vi "GCOMM Close.vi"(8 "error in":errorcluster, 11 "session in":T1) -> (0 "error out":errorcluster, 3 "session out":T1)   [LabVIEW 2013]
doc: "Opens generic COM port multiplexer."
uses:
  GCOMM Session.ctl
  GCOMM Signal.ctl
  GCOMM Virtual Channel.ctl
  GCOMM Logic State.ctl
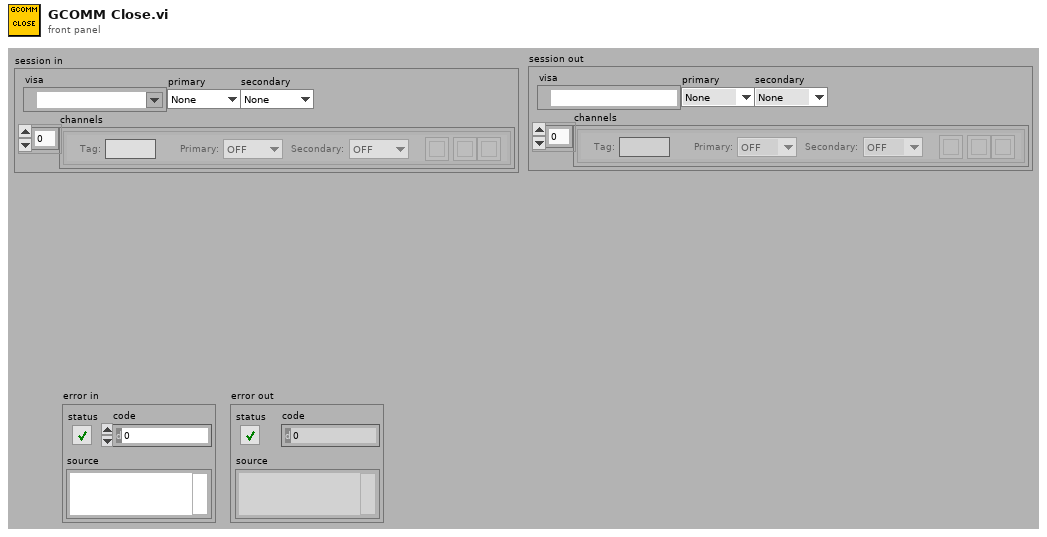
[diagram p1: front panel]
types:
  T1 = typedef "GCOMM Session.ctl" = cluster{"visa":refnum<visa-resource-name>, "primary":T2, "secondary":T2, "channels":T3[]}
  T2 = typedef "GCOMM Signal.ctl" = enum16{"None", "DTR", "RTS"}
  T3 = typedef "GCOMM Virtual Channel.ctl" = cluster{"Primary:":T4, "Secondary:":T4, "btn clr":bool, "btn up":bool, "btn down":bool, "Tag:":string}
  T4 = typedef "GCOMM Logic State.ctl" = enum16{"OFF", "ON"}
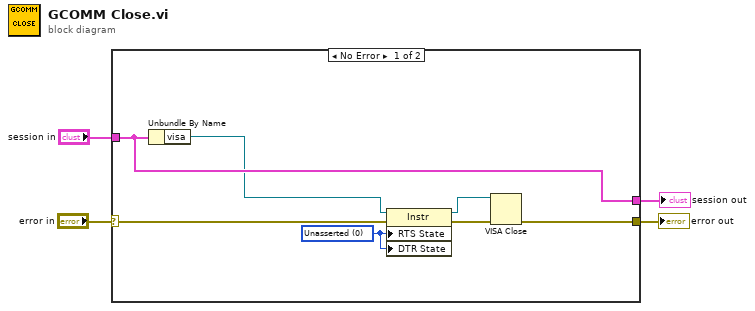
[diagram p0: block diagram]
diagram:
  n1 = case shown="No Error" "error in" {
    selector: "error in" -> [w6 w13]
    tunnel: [w11 w13] -> w4
    tunnel: "session in" -> [w10 w12]
    tunnel: [w10 w12] -> w2
    frame No Error {
      w5 = i16 0 items=["Unknown"=-1, "Unasserted"=0, "Asserted"=1] ("Serial Settings:Modem Line Settings:Line RTS State")
      n2 = Unbundle By Name(w10) -> ("visa"=w8:refnum<visa-resource-name>)
      n3 = property class="Instr"(reference=w8, error in=w6, "RTS State"=w5, "DTR State"=w5) -> (reference out=w7:refnum<visa-resource-name>, error out=w9:errorcluster)
      n4 = VISA Close(VISA resource name=w7, error in (no error)=w9) -> (error out=w11:errorcluster)
    }
    frame Error {
    }
  }
  "error out" <- w4
  "session out" <- w2
